vi "Remove Waveform in List.vi"(7 "Waveform List Ctl Ref":refnum<vi>, 8 "error in (no error)":errorcluster, 11 "Canvas Wfm Array In":waveform(dbl)[](array[waveform])) -> (0 "error out":errorcluster, 3 "Canvas Wfm Array Out":waveform(dbl)[](array[waveform]))   [LabVIEW 2025, in "TDMS Waveform Creator UI.lvlib"]
uses:
  TDMS Waveform Creator UI.lvlib
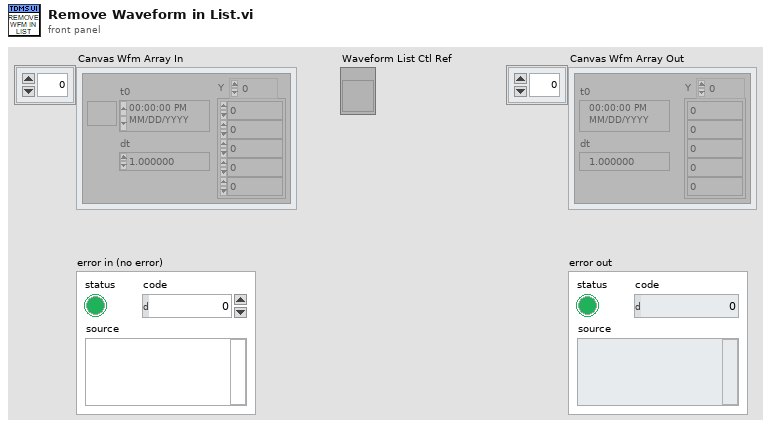
[diagram p1: front panel]
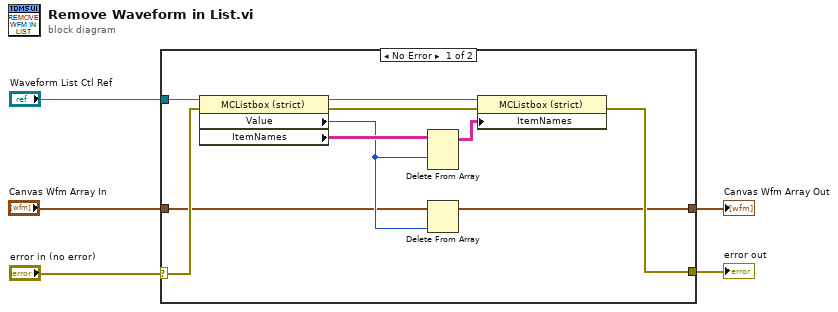
[diagram p0: block diagram]
diagram:
  n1 = case shown="No Error" "error in (no error)" {
    selector: "error in (no error)" -> [w13 w17]
    tunnel: "Waveform List Ctl Ref" -> [w15 _]
    tunnel: "Canvas Wfm Array In" -> [w6 w16]
    tunnel: [w9 w16] -> w2
    tunnel: [w12 w17] -> w1
    frame No Error {
      n2 = property class="MCListbox (strict)"(reference=w15, error in=w13) -> (reference out=w14:refnum<vi>, error out=w11:errorcluster, "Value"=w7:i32, "ItemNames"=w10:string[][])
      n3 = Delete From Array(array=w10, index (row)=w7) -> (array with subset deleted=w8:string[][])  [unwired: 2 in, 1 out]
      n4 = Delete From Array(array=w6, index=w7) -> (array with subset deleted=w9:waveform(dbl)[])  [unwired: 1 in, 1 out]
      n5 = property class="MCListbox (strict)"(reference=w14, error in=w11, "ItemNames"=w8) -> (error out=w12:errorcluster)  [unwired: 1 out]
    }
    frame Error {
    }
  }
  "error out" <- w1
  "Canvas Wfm Array Out" <- w2
